vi "XY Go.vi"(8 "error in (no error)":errorcluster, 9 "Speed":dbl, 10 "XY":dbl[](array[numeric]), 11 "Gantry In":refnum<k24>) -> (0 "error out":errorcluster, 3 "Gantry Out":refnum<k24>)   [LabVIEW 2019, in "A3200.lvclass"]
uses:
  A3200.lvclass
  C:/Program Files (x86)/Aerotech/A3200/LabVIEW/2010/Bin/Aerotech.A3200.dll
  Program Files (x86)/Aerotech/A3200/LabVIEW/2010/Bin/Aerotech.A3200.dll
  Drivers/Aerotech A3200/Aerotech VIs.lvlib
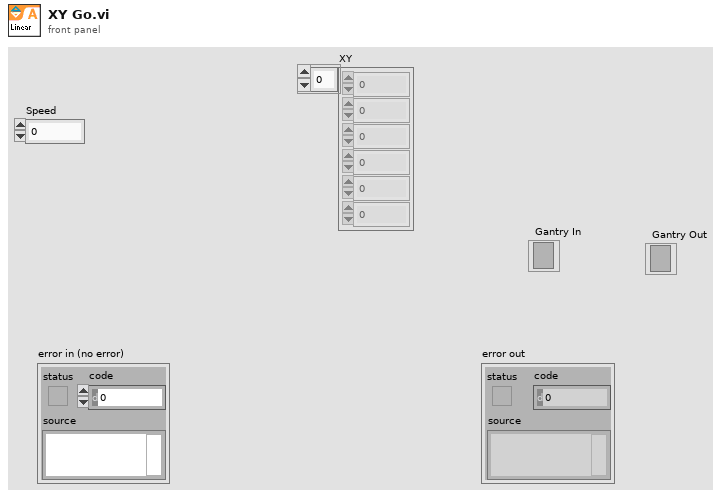
[diagram p1: front panel]
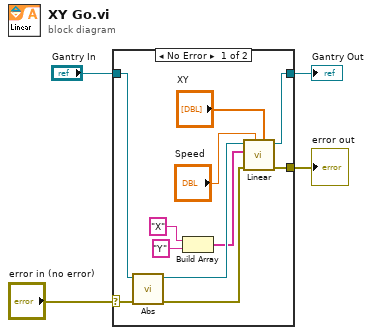
[diagram p0: block diagram]
diagram:
  n1 = case shown="No Error" "error in (no error)" {
    selector: "error in (no error)" -> [w9 w17]
    tunnel: [w6 w17] -> w3
    tunnel: "Gantry In" -> [w10 w16]
    tunnel: [w5 w16] -> w1
    frame No Error {
      n2 = call "Abs.vi"("error in (no error)"=w9, "controller in"=w10) -> ("error out"=w8:errorcluster, "controller out"=w12:refnum<k24>)  [unwired: 8 in]
      n3 = Build Array("X" ("format string"), "Y" ("format string")) -> (w7:string[])
      n4 = call "Linear.vi"("distances"="XY", "speed"="Speed", "error in (no error)"=w8, "axis names"=w7, "controller in"=w12) -> ("error out"=w6:errorcluster, "controller out"=w5:refnum<k24>)  [unwired: 5 in]
    }
    frame Error {
    }
  }
  "error out" <- w3
  "Gantry Out" <- w1
